vi "String Ctl Cursor to End.vi"(8 "error in (no error)":errorcluster, 11 "String Reference in":refnum<vi>) -> (0 "error out":errorcluster)   [LabVIEW 2012]
doc: "SciScan 1.2 160622\nSets key focus to string control and moves cursor to end of string"
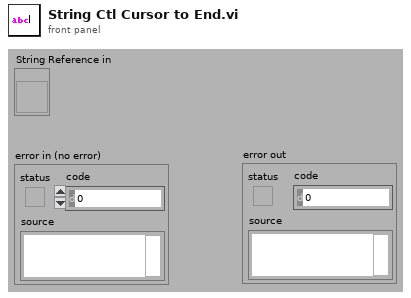
[diagram p1: front panel]
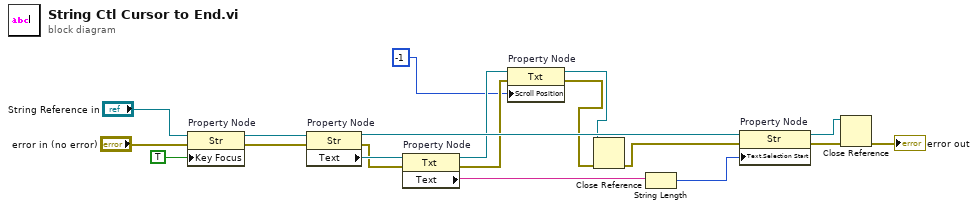
[diagram p0: block diagram]
diagram:
  n1 = property on="Property Node" class="Str"(reference="String Reference in", error in="error in (no error)", "Key Focus"=TRUE) -> (reference out=w17:refnum<vi>, error out=w16:errorcluster)
  n2 = property on="Property Node" class="Str"(reference=w17, error in=w16) -> (reference out=w13:refnum<vi>, error out=w15:errorcluster, "Text"=w18:refnum<vi>)
  n3 = property on="Property Node" class="Txt"(reference=w18, error in=w15) -> (reference out=w3:refnum<vi>, error out=w5:errorcluster, "Text"=w12:string)
  n4 = property on="Property Node" class="Txt"(reference=w3, error in=w5, "Scroll Position"=-1) -> (reference out=w2:refnum<vi>, error out=w4:errorcluster)
  n5 = Close Reference(reference=w2, error in (no error)=w4) -> (error out=w9:errorcluster)
  n6 = String Length(string=w12) -> (length=w11:i32)
  n7 = property on="Property Node" class="Str"(reference=w13, error in=w9, "Text.Selection Start"=w11) -> (reference out=w8:refnum<vi>, error out=w7:errorcluster)
  n8 = Close Reference(reference=w8, error in (no error)=w7) -> (error out=→"error out":errorcluster)
